vi "KB-CalColorOrExist.vi"(8 "error in (no error)":errorcluster, 9 "y":i32=300, 10 "ROI Descriptor":T2={"Global Rectangle"=[-1, -1, 2, 2], "Contours"=[{"ID"=enum."External", "Type"=7, "Coordinates"=[0, 0, 0, 0, 0, 0]}]} {"Contours"."Type" items=["No Selection", "Point", "Line", "Rectangle", "Oval", "Polygon", "Freehand Region", "Annulus", "Unused2", "Unused3", "Broken Line", "Freehand Line", "Rotated Rectangle"]}, 11 "Image In":T3(plugin-control)) -> (0 "error out":errorcluster, 1 "漏装结果":string, 2 "颜色结果":string, 3 "Image Out":T3(plugin-control), 4 "白色和金色":i32)   [LabVIEW 2015]
uses:
  <vilib>/vision/NI_Vision_Development_Module.lvlib
panel:
  out "Pixel Value (U64)":T1
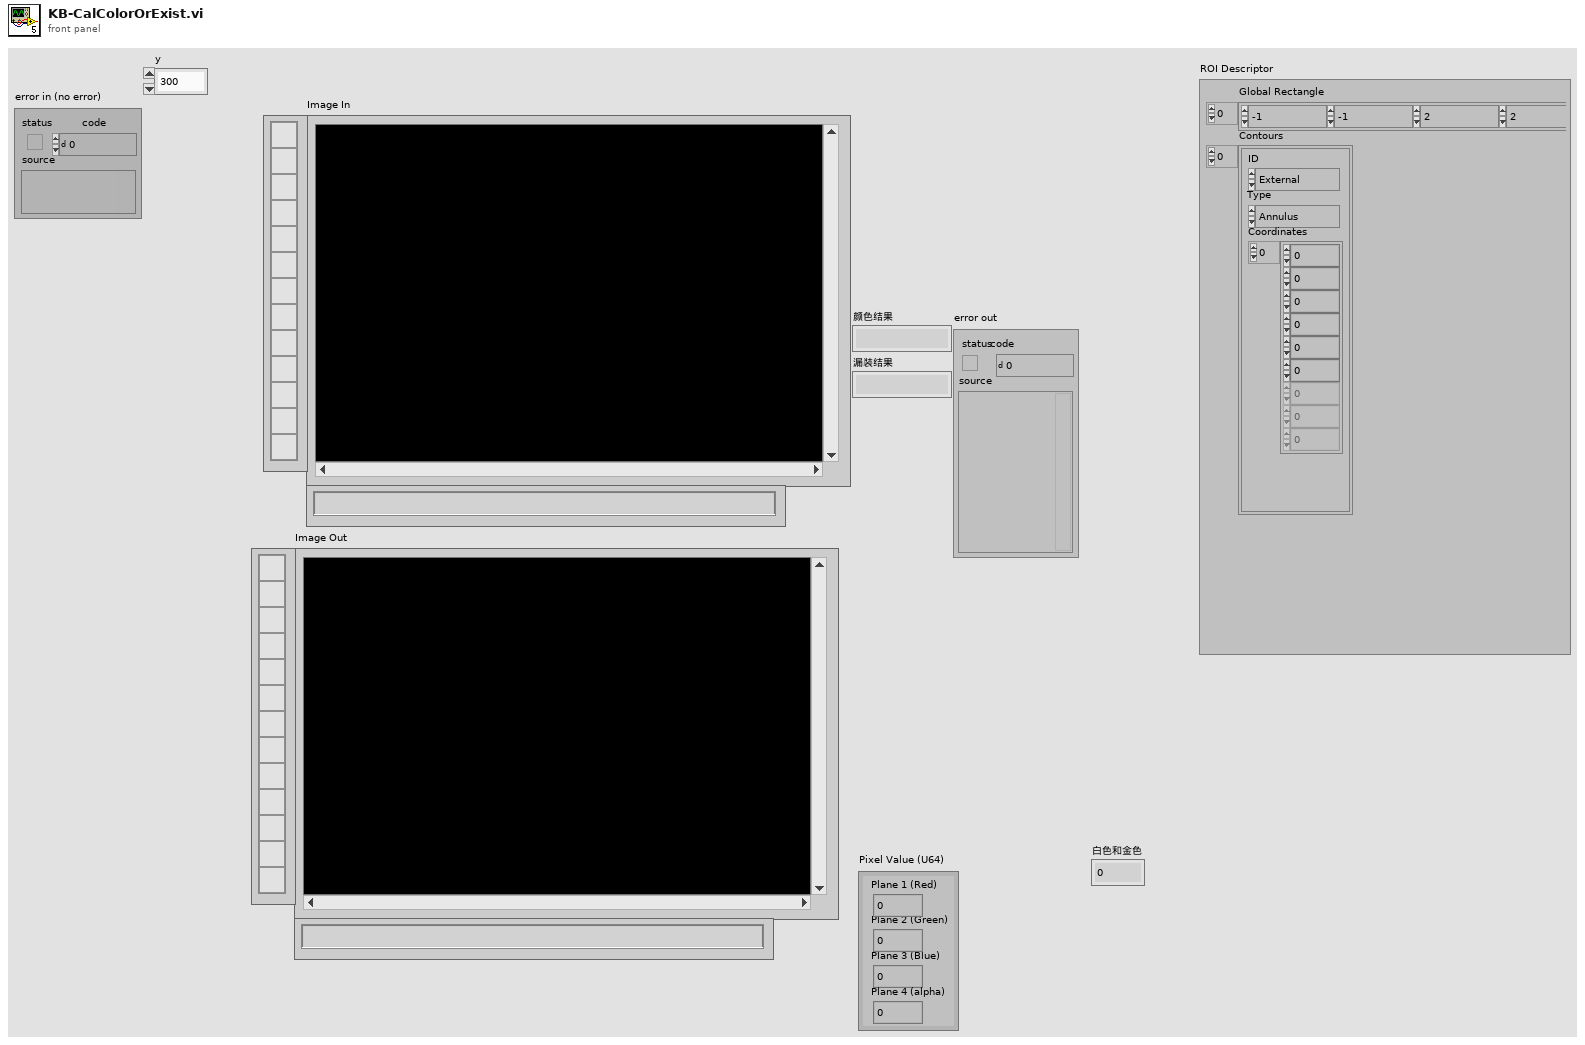
[diagram p1: front panel]
types:
  T1 = typedef "Color (U64)" = cluster{"Plane 3 (Blue)":u16, "Plane 2 (Green)":u16, "Plane 1 (Red)":u16, "Plane 4 (alpha)":u16}
  T2 = typedef "ROI Descriptor" = cluster{"Global Rectangle":i32[], "Contours":cluster{"ID":enum32{"External", "Internal"}, "Type":u32, "Coordinates":i32[]}[]}
  T3 = typedef "IMAQ Image.ctl" = refnum<image>
  T4 = typedef "Image Type" = u32
  T5 = typedef "IMAQ Point" = cluster{"X":sgl, "Y":sgl}
  T6 = cluster{"Red (or Hue) value":u8, "Green (or Sat) value":u8, "Blue (or Light or Val) value":u8}
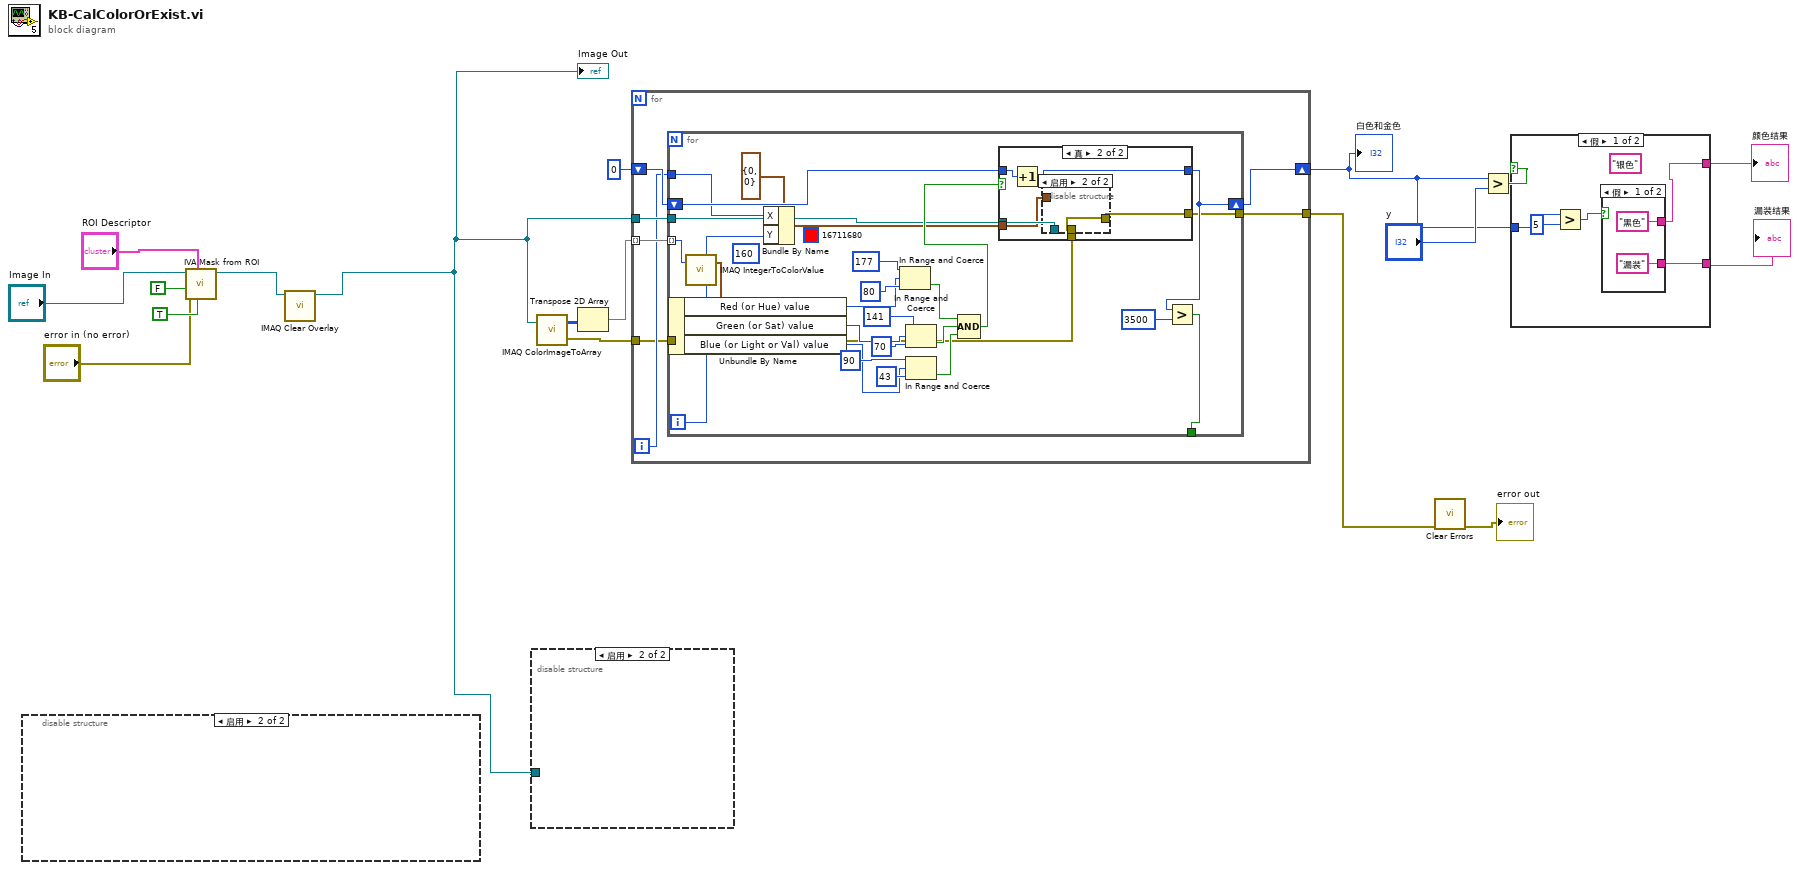
[diagram p0: block diagram]
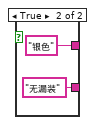
[diagram p2: hidden frame]
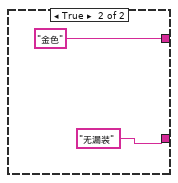
[diagram p3: hidden frame]
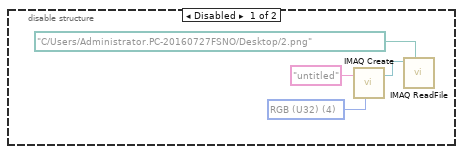
[diagram p4: hidden frame]
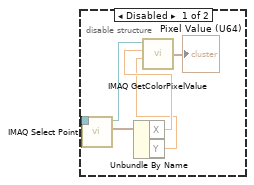
[diagram p5: hidden frame]
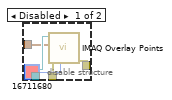
[diagram p7: hidden frame]
diagram:
  n1 = disable-structure shown="启用" {
    frame Disabled {
      w19 = T4 4 items=["Grayscale (U8)", "Grayscale (I16)", "Grayscale (SGL)", "Complex (CSG)", "RGB (U32)", "HSL (U32)", "RGB (U64)", "Grayscale (U16)"] ("Image Type")
      n2 = call "IMAQ Create"("Image Name"="untitled", "Image Type"=w19) -> ("New Image"=w21:T3)  [unwired: 3 in, 1 out]
      n3 = call "IMAQ ReadFile"("File Path"=path "C:/Users/Administrator.PC-20160727FSNO/Desktop/2.png", "Image"=w21) -> ()  [unwired: 5 in, 5 out]
    }
    frame Enabled {
    }
  }
  n4 = call <vilib>:"IVA Mask from ROI.vi"("Shrink"=TRUE, "ROI Descriptor"="ROI Descriptor", "error in (no error)"="error in (no error)", "Out / In"=FALSE, "Image Src"="Image In") -> ("Image Out"=w6:T3)  [unwired: 6 out]
  n5 = call "IMAQ Clear Overlay"("Image"=w6) -> ("Image Out"=w1:T3)  [unwired: 9 in, 1 out]
  "Image Out" <- w1
  n6 = disable-structure shown="启用" {
    disable-tunnel: w1 -> [w28 _]
    frame Disabled {
      n7 = call "IMAQ Select Point"("Image In"=w28) -> ("Point"=w26:T5, "Image Out (duplicate)"=w27:T3)  [unwired: 7 in, 2 out]
      n8 = Unbundle By Name(w26) -> ("X"=w25:sgl, "Y"=w24:sgl)
      n9 = call "IMAQ GetColorPixelValue"("Y Coordinate"=w24, "X Coordinate"=w25, "Image"=w27) -> ("Pixel Value (U64)"=→"Pixel Value (U64)":T1)  [unwired: 1 in, 2 out]
    }
    frame Enabled {
    }
  }
  n10 = call "IMAQ ColorImageToArray"("Image"=w1) -> ("Image Pixels (U32)"=w3:u32[][], "error out"=w5:errorcluster)  [unwired: 3 in, 1 out]
  n11 = Transpose 2D Array(2D array=w3) -> (transposed array=w2:u32[][])
  n12 = for {
    tunnel: w2 -> [w35] mode=indexing
    shift-right: [w33] -> w8
    shift-left: 0 -> [w34]
    tunnel: w1 -> [w32]
    tunnel: w5 -> [w30]
    tunnel: [w29] -> w4
    i -> [w31]
    n13 = for {
      tunnel: w35 -> [w59] mode=indexing
      shift-right: [w45] -> w33
      shift-left: w34 -> [w60]
      tunnel: [w36] -> _
      tunnel: w32 -> [w42]
      tunnel: w31 -> [w37]
      tunnel: w30 -> [w40]
      tunnel: [w39] -> w29
      i -> [w38]
      (unwired) u32 16711680 ("Color")
      (unwired) u8 160 ("下限")
      n14 = call "IMAQ IntegerToColorValue"("U32 value"=w59) -> ("Color Value"=w58:T6)  [unwired: 4 in, 3 out]
      n15 = Unbundle By Name(w58) -> ("Red (or Hue) value"=w52:u8, "Green (or Sat) value"=w51:u8, "Blue (or Light or Val) value"=w50:u8)
      n16 = Bundle By Name(cluster=cluster{"X":i32, "Y":i32} {"X"=0, "Y"=0} ("Point"), "X"=w37, "Y"=w38) -> (w41:cluster{"X":i32, "Y":i32})
      n17 = In Range and Coerce(upper limit=u8 177 ("上限"), x=w52, lower limit=u8 80 ("下限")) -> (In Range?=w49:bool)  [unwired: 1 out]
      n18 = In Range and Coerce(upper limit=u8 141 ("上限"), x=w51, lower limit=u8 70 ("下限")) -> (In Range?=w48:bool)  [unwired: 1 out]
      n19 = In Range and Coerce(upper limit=u8 90 ("上限"), x=w50, lower limit=u8 43 ("下限")) -> (In Range?=w47:bool)  [unwired: 1 out]
      n20 = Compound Arithmetic op=AND ("复合运算")(w49, w48, w47) -> (w46:bool)
      n21 = case shown="真" w46 {
        tunnel: w60 -> [w63 w69]
        tunnel: [w63 w68] -> w45
        tunnel: w42 -> [_ w67]
        tunnel: w41 -> [_ w66]
        tunnel: w40 -> [w62 w65]
        tunnel: [w62 w64] -> w39
        frame False {
        }
        frame True {
          n22 = Increment(x=w69) -> (x+1=w68:i32)
          n23 = disable-structure shown="启用" {
            disable-tunnel: w67 -> [w74 _]
            disable-tunnel: w66 -> [w73 _]
            disable-tunnel: w65 -> [w71 w75]
            disable-tunnel: [w70 w75] -> w64
            frame Disabled {
              n24 = call "IMAQ Overlay Points"("Color"=u32 16711680, "error in (no error)"=w71, "Point"=w73, "Image"=w74) -> ("error out"=w70:errorcluster)  [unwired: 6 in, 1 out]
            }
            frame Enabled {
            }
          }
        }
      }
      n25 = Greater?(x=w45, y=3500) -> (0:w36:bool)
    }
  }
  "白色和金色" <- w8
  n26 = call <vilib>:"Clear Errors.vi"("error in (no error)"=w4) -> ("error out"=→"error out":errorcluster)  [unwired: 5 in, 1 out]
  n27 = Greater?(x=w8, y="y") -> (0:w9:bool)
  n28 = case shown="假" w9 {
    tunnel: [w79 "金色"] -> w15
    tunnel: w8 -> [w77 _]
    tunnel: [w78 "无漏装"] -> w7
    frame False {
      (unwired) "银色"
      n29 = Greater?(x=w77, y=5) -> (0:w80:bool)
      n30 = case shown="假" w80 {
        tunnel: ["黑色" "银色"] -> w79
        tunnel: ["漏装" "无漏装"] -> w78
        frame False {
        }
        frame True {
        }
      }
    }
    frame True {
    }
  }
  "颜色结果" <- w15
  "漏装结果" <- w7
